vi "available modifications.vi"() -> ()   [LabVIEW 2013, in "VI modification collection.lvclass"]
uses:
  VI modification collection.lvclass
  VI modification.lvclass
panel:
  in  "available mods":refnum<class "VI modification.lvclass">[](array[class])
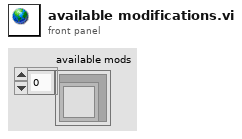
[diagram p1: front panel]
diagram:
